vi "Remove Spaces From String.vi"(11 "String in":string=" a b c d e f ") -> (3 "string":string)   [LabVIEW 2020, in "ADAS_IO_Template_MDO.lvclass"]
uses:
  ADAS_IO_Template_MDO.lvclass
  ADAS_IO_Template_MDO.lvclass/ADAS_IO_Template_MDO.ctl
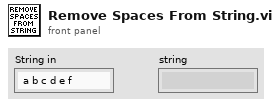
[diagram p1: front panel]
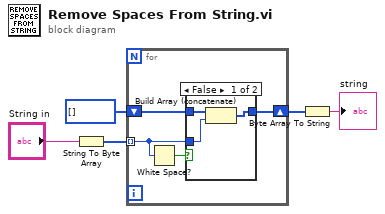
[diagram p0: block diagram]
diagram:
  n1 = String To Byte Array(string="String in") -> (unsigned byte array=w5:u8[])
  n2 = for {
    tunnel: w5 -> [w8] mode=indexing
    shift-right: [w6] -> w3
    shift-left: u8[] [] ("unsigned byte array") -> [w7]
    n3 = White Space?(1:w8) -> (0:w9:bool)
    n4 = case shown="False" w9 {
      tunnel: w8 -> [w11 _]
      tunnel: w7 -> [w12 w13]
      tunnel: [w10 w13] -> w6
      frame False {
        n5 = Build Array (concatenate)(w12, w11) -> (w10:u8[])
      }
      frame True {
      }
    }
  }
  n6 = Byte Array To String(unsigned byte array=w3) -> (string=→"string":string)
